vi "Find Next Timestamp.vi"(8 "error in (no error)":errorcluster, 11 "Monthly in":refnum<class "Monthly.lvclass">) -> (0 "error out":errorcluster, 3 "Monthly out":refnum<class "Monthly.lvclass">)   [LabVIEW 2020, in "Monthly.lvclass"]
uses:
  Monthly.lvclass
  Monthly.lvclass/Monthly.ctl
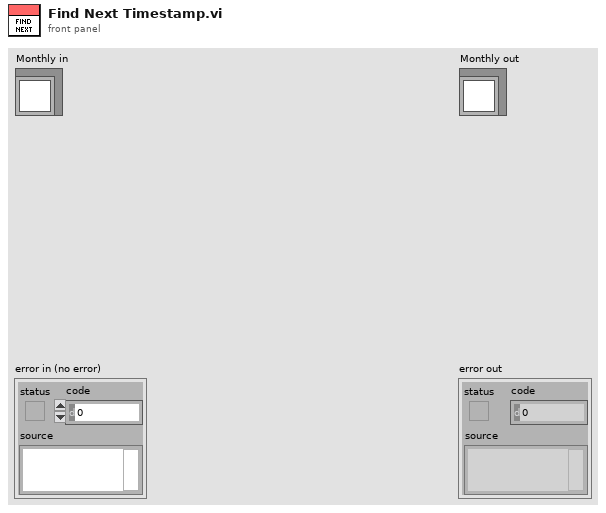
[diagram p1: front panel]
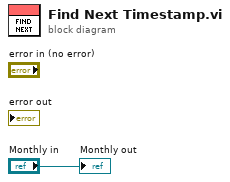
[diagram p0: block diagram]
diagram:
  "Monthly out" <- "Monthly in"
